vi "TopicRequest_Respond.vi"(3 "port":u16, 4 "XML":string, 5 "Subscribers":T2(array[cluster])) -> (1 "Topic Request Reply":string, 2 "Subscribers":T2(array[cluster]))   [LabVIEW 2013]
panel:
  out "New Subscriber":T1
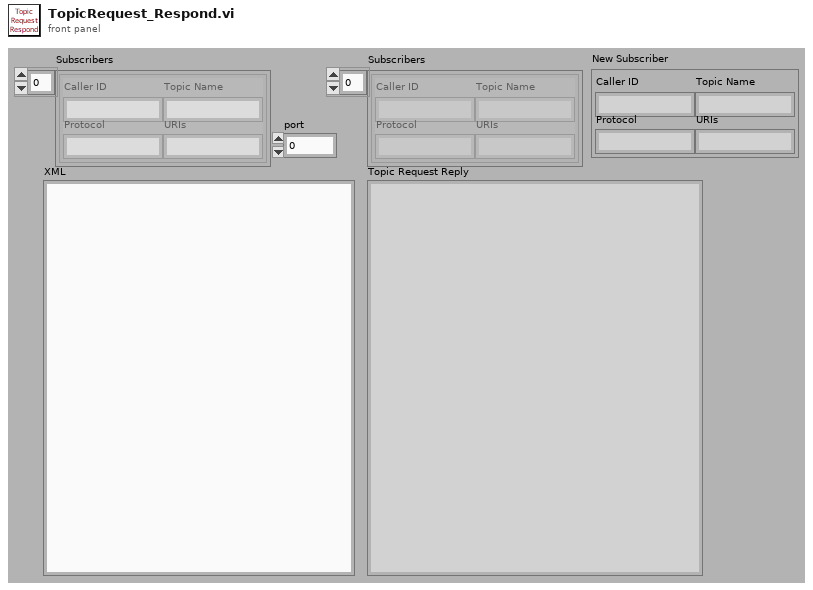
[diagram p1: front panel]
types:
  T1 = cluster{"Caller ID":string, "Topic Name":string, "Protocol":string, "URIs":string}
  T2 = cluster{"Caller ID":string, "Topic Name":string, "Protocol":string, "URIs":string}[]
  T3 = enum16{"http://IP:port", "http://IP", "IP:port", "IP only"}
  T4 = cluster{"Caller ID":string, "Topic Name":string, "Protocol":string, "URI":string}
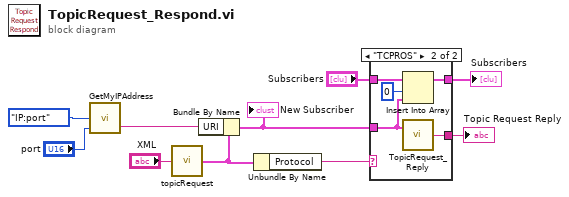
[diagram p0: block diagram]
diagram:
  n1 = call "GetMyIPAddress.vi"("Port"="port", "Format"=T3."IP:port") -> ("URI"=w2:string)  [unwired: 2 in]
  n2 = call "topicRequest.vi"("XML"="XML") -> ("Subscriber"=w5:T4)
  n3 = Bundle By Name(cluster=w5, "URI"=w2) -> (w1:T4)
  "New Subscriber" <- w1
  n4 = Unbundle By Name(w5) -> ("Protocol"=w9:string)
  n5 = case shown="\"TCPROS\"" w9 {
    tunnel: "Subscribers" -> [w11 w16]
    tunnel: w1 -> [_ w12]
    tunnel: [w11 w15] -> w6
    tunnel: [_ w14] -> w8
    frame "False", Default {
    }
    frame "TCPROS" {
      n6 = Insert Into Array(array=w16, index=0, new element=w12) -> (w15:T2)
      n7 = call "TopicRequest_Reply.vi"("New Subscriber"=w12) -> ("XML"=w14:string)  [unwired: 1 in]
    }
  }
  "Subscribers" <- w6
  "Topic Request Reply" <- w8
